vi "insert_edge.vi"(10 "edge":refnum<class "Edge.lvclass">, 11 "digraph":refnum<class "DiGraph.lvclass">) -> (1 "edge unchanged?":bool, 2 "edge already included?":bool, 3 "digraph out":refnum<class "DiGraph.lvclass">)   [LabVIEW 2020, in "graph.lvlib" / "DiGraph.lvclass"]
uses:
  DiGraph.lvclass
  Edge/Edge.lvclass
  DiGraph.lvclass/DiGraph.ctl
  192cd781-888a-4283-9972-3738ebc0cdeb.vi
  4775521a-dcdb-4985-b41c-6a23402e0cd2.vi
  Graph/Graph.lvclass
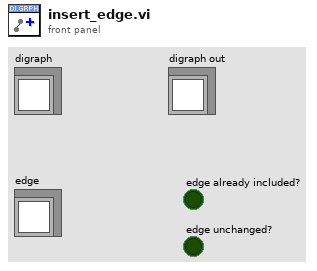
[diagram p1: front panel]
types:
  T1 = map{refnum<class "ID.lvclass">, set{refnum<class "ID.lvclass">}}
  T2 = typedef "edge-definition-cluster.ctl" = cluster{"source-id":refnum<class "ID.lvclass">, "sink-id":refnum<class "ID.lvclass">}
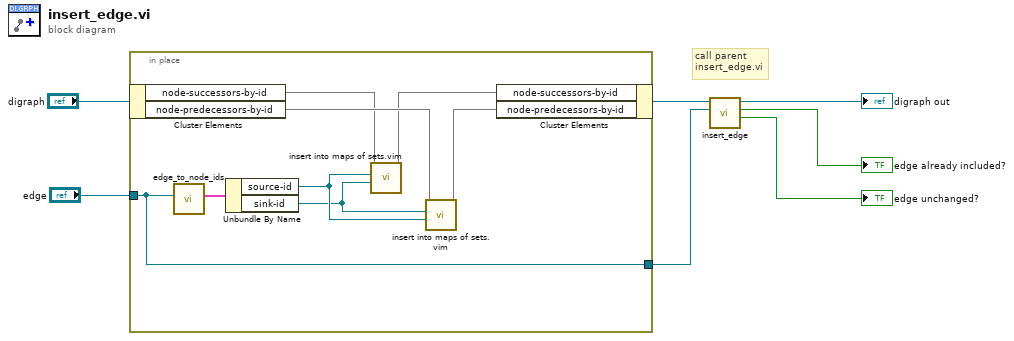
[diagram p0: block diagram]
diagram:
  # "call parent\ninsert_edge.vi"
  n1 = in-place {
    in-place-border: "edge" -> [w8]
    in-place-border: [w8] -> w3
    n2 = in-place-cluster #1("digraph") -> ("node-successors-by-id"=w14:T1, "node-predecessors-by-id"=w15:T1)
    n3 = call "edge_to_node_ids.vi"("edge"=w8) -> ("node-ids-cluster"=w9:T2)  [unwired: 10 in]
    n4 = Unbundle By Name(w9) -> ("source-id"=w11:refnum<class "ID.lvclass">, "sink-id"=w10:refnum<class "ID.lvclass">)
    n5 = call "insert into maps of sets.vim"("value"=w10, "key"=w11, "map of sets in"=w14) -> ("map of sets out"=w13:T1)  [unwired: 8 in]
    n6 = call "insert into maps of sets.vim"("value"=w11, "key"=w10, "map of sets in"=w15) -> ("map of sets out"=w12:T1)  [unwired: 8 in]
    n7 = in-place-cluster #1("node-successors-by-id"=w13, "node-predecessors-by-id"=w12) -> (w5:refnum<class "DiGraph.lvclass">)
  }
  n8 = call-parent "insert_edge.vi"("edge"=w3, "digraph"=w5) -> ("edge unchanged?"=→"edge unchanged?":bool, "edge already included?"=→"edge already included?":bool, "digraph out"=→"digraph out":refnum<class "DiGraph.lvclass">)  [unwired: 7 in]
